vi "DelayGenerator-CentralCarriage.vi"(3 "Time Stamp":timestamp, 9 "error in (no error)":errorcluster caption="error out") -> (0 "DelayTarget":T1, 6 "error out":errorcluster)   [LabVIEW 2009]
uses:
  Controls/DelayTarget.ctl
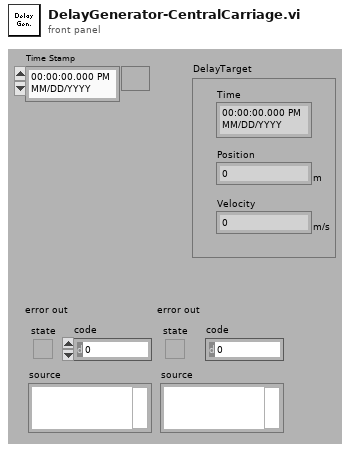
[diagram p1: front panel]
types:
  T1 = typedef "DelayTarget.ctl" = cluster{"Time":timestamp, "Position":dbl[unit], "Velocity":dbl[unit]}
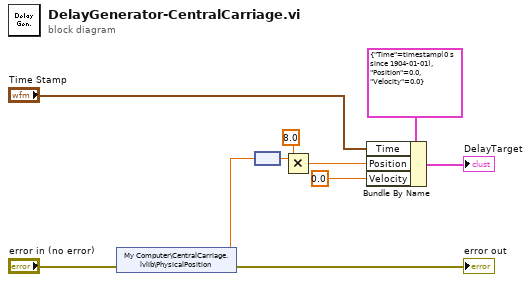
[diagram p0: block diagram]
diagram:
  n1 = shared-variable "My Computer\\CentralCarriage.lvlib\\PhysicalPosition"(error in="error in (no error)") -> (w2:dbl, error out=→"error out":errorcluster)
  n2 = node(w2) -> (w1:dbl[unit])
  n3 = Multiply(x=w1, y=8.0) -> (x*y=w7:dbl[unit])
  n4 = Bundle By Name(cluster=T1 {"Time"=timestamp(0 s since 1904-01-01), "Position"=0.0, "Velocity"=0.0} ("DelayTarget"), "Time"="Time Stamp", "Position"=w7, "Velocity"=dbl[unit] 0.0) -> (→"DelayTarget":T1)
